vi "Generate_Voice_Event.vi"(8 "Error In":errorcluster, 11 "Voice Control Reference In":T1) -> (0 "Error Out":errorcluster, 3 "Voice Control Reference Out":T1)   [LabVIEW 2018]
uses:
  Data Def/Voice Control Reference.ctl
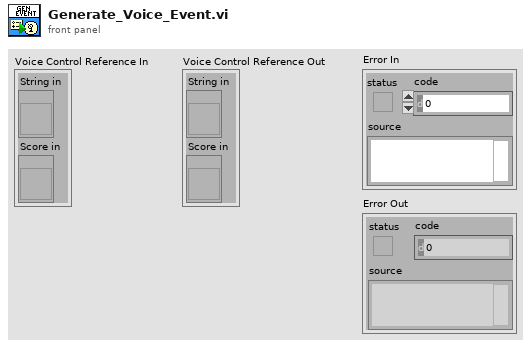
[diagram p1: front panel]
types:
  T1 = typedef "Voice Control Reference.ctl" = cluster{"String in":refnum<vi>, "Score in":refnum<vi>}
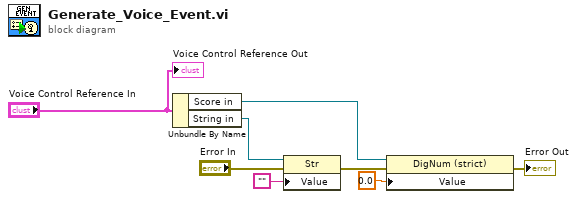
[diagram p0: block diagram]
diagram:
  n1 = Unbundle By Name("Voice Control Reference In") -> ("Score in"=w4:refnum<vi>, "String in"=w8:refnum<vi>)
  n2 = property class="Str"(reference=w8, error in="Error In", "Value"="") -> (error out=w5:errorcluster)  [unwired: 1 out]
  n3 = property class="DigNum (strict)"(reference=w4, error in=w5, "Value"=0.0) -> (error out=→"Error Out":errorcluster)  [unwired: 1 out]
  "Voice Control Reference Out" <- "Voice Control Reference In"
